vi "Temperatures.vi"(1 "Update Interval":i32=2 min=0 max=600, 2 "Control\nTemperature":sgl=-200.0 format="%.1f") -> (0 "DiodeTemp":dbl(slide) scale=-150.0..50.0)   [LabVIEW 2014]
uses:
  DetectorGlobals.vi
panel:
  in  "Tab Control":enum32{"CamTemp", "DewTemp", "Diode", "Temp4"}(tab)
  out "CamTemp Chart":dbl(graph)
  out "DewTemp Chart":dbl(graph)
  out "Diode Chart":dbl(graph)
  out "Temp4 Chart":dbl(graph)
  out "Utility Board\nInstalled":bool
  out "Temp 4":dbl(slide) scale=-150.0..50.0
  in  "Read Temps":bool
  out "Time1":dbl format="%.2f"
  out "refnum":refnum<file>
  in  "Log Data":bool
  in  "Read Heater":bool=TRUE caption="Read"
  out "Heater\nPower":dbl(knob) scale=0.0..3072.0
  out "DewTemp":dbl(slide) scale=-200.0..50.0
  out "CamTemp":dbl(slide) scale=-150.0..50.0
  in  "Set":bool
  # "C"
  # "sec"
  # "Degrees Celsius"
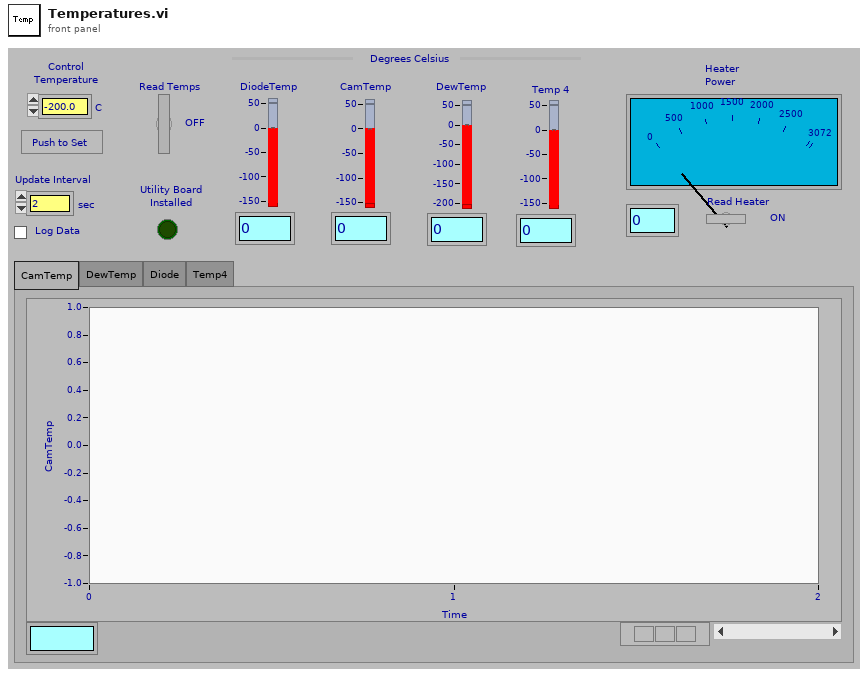
[diagram p1: front panel]
types:
  T1 = enum32{"not used", "PCI_BOARD", "TIMING_BOARD", "UTILITY_BOARD"}
  T2 = enum16{"open", "open or create", "create or replace", "create", "open (read only)"}
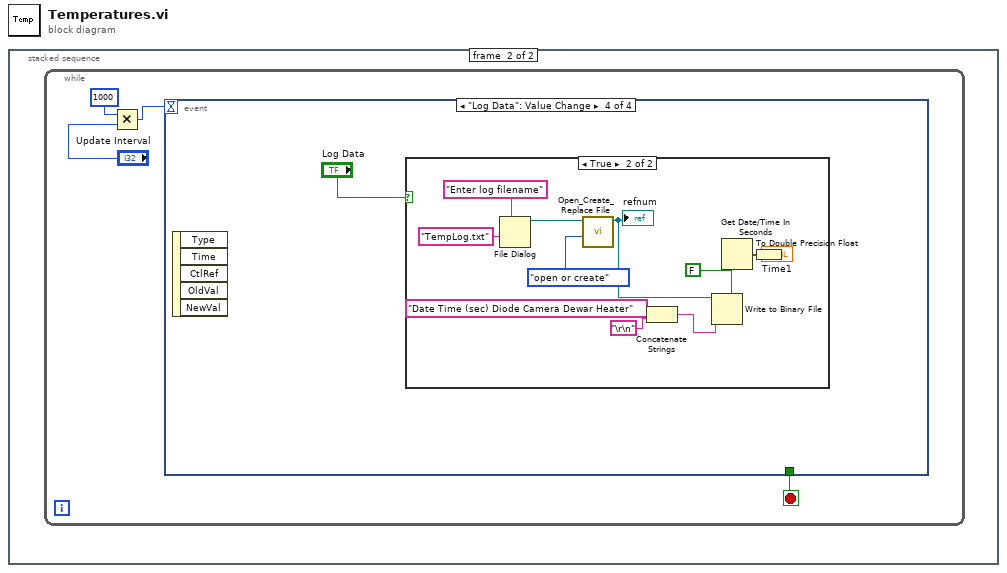
[diagram p0: block diagram]
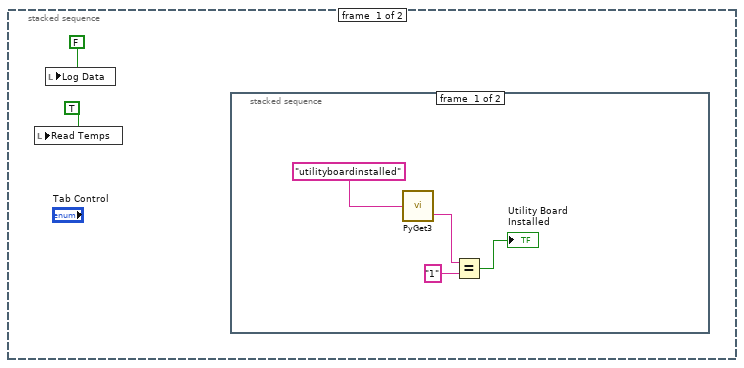
[diagram p2: hidden frame]
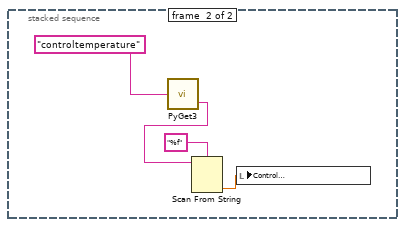
[diagram p3: hidden frame]
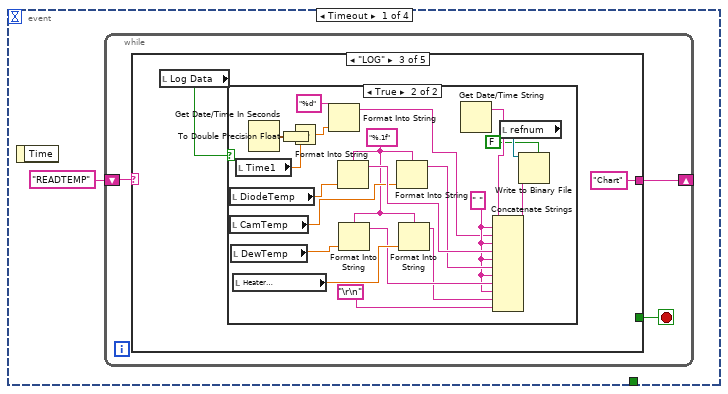
[diagram p4: hidden frame]
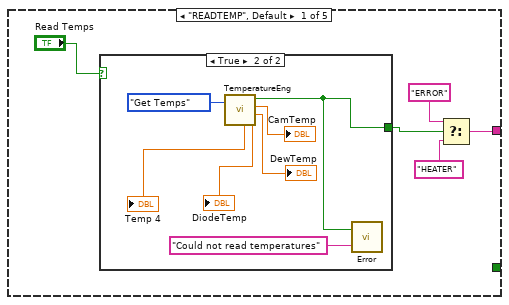
[diagram p5: hidden frame]
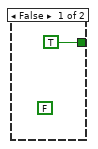
[diagram p6: hidden frame]
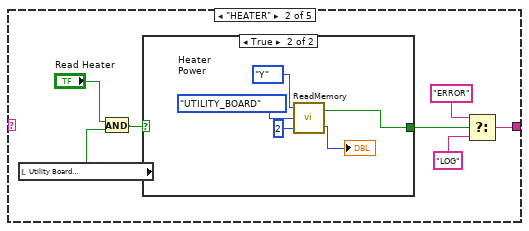
[diagram p7: hidden frame]
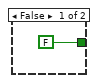
[diagram p8: hidden frame]
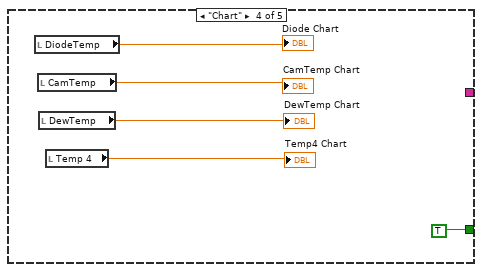
[diagram p10: hidden frame]
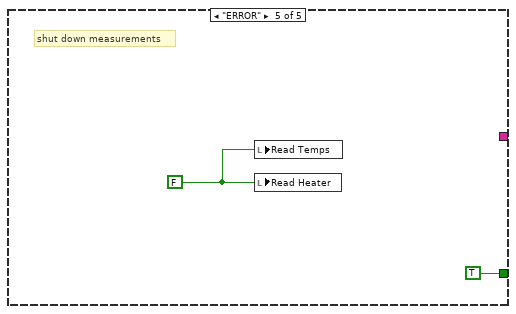
[diagram p11: hidden frame]
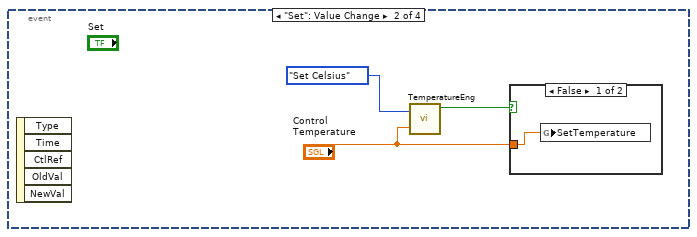
[diagram p12: hidden frame]
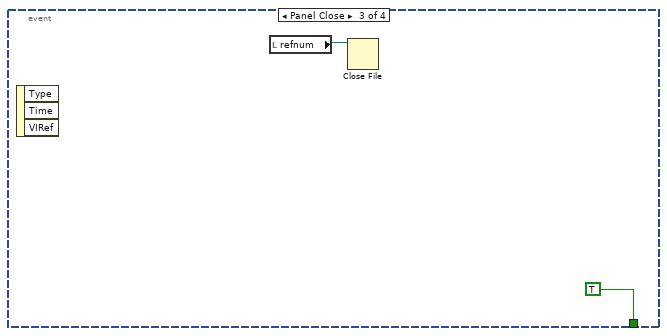
[diagram p14: hidden frame]
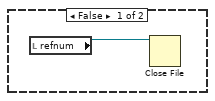
[diagram p15: hidden frame]
diagram:
  n1 = stacked-sequence {
    frame #0 {
      n2 = local write "Read Temps"(TRUE ("ReadTemps")) -> ()
      n3 = local write "Log Data"(FALSE ("Log Data")) -> ()
      n4 = stacked-sequence {
        frame #0 {
          n5 = call "PyGet3.vi"("Attribute"="utilityboardinstalled") -> ("Reply"=w5:string)  [unwired: 1 out]
          n6 = Equal?(x=w5, y="1") -> (x = y?=→"Utility Board\nInstalled":bool)
        }
        frame #1 {
          n7 = call "PyGet3.vi"("Attribute"="controltemperature") -> ("Reply"=w9:string)  [unwired: 1 out]
          n8 = Scan From String(format string="%f", input string=w9) -> (output 1=w7:dbl)  [unwired: 3 in, 3 out]
          n9 = local write "Control\nTemperature"(w7) -> ()
        }
      }
    }
    frame #1 {
      n10 = while {
        stop <- w11 stop-if-true
        n11 = Multiply(x=1000, y="Update Interval") -> (x*y=w13:i32)
        n12 = event shown="[3] \"Log Data\": Value Change" {
          selector: _ -> [_ _ _ _]
          dyn-events: _ -> [_ _ _ _]
          timeout: w13 -> [_ _ _ _]
          tunnel: [_ _ TRUE _] -> w11
          event Timeout {
            n13 = event-data() -> ()  [unwired: 1 in, 1 out]
            n14 = while {
              shift-right: [w18] -> _
              shift-left: "READTEMP" ("Error String") -> [w17]
              stop <- w16 stop-if-true
              n15 = case shown="\"LOG\"" w17 {
                tunnel: [w23 w38 "Chart" ("Error String") _ _] -> w18
                tunnel: [_ _ _ TRUE TRUE] -> w16
                frame "READTEMP", Default {
                  n16 = case shown="True" "Read Temps" {
                    tunnel: [TRUE w30] -> w22
                    frame False {
                      (unwired) FALSE ("Error")
                    }
                    frame True {
                      n17 = call "TemperatureEng.vi"("Action"=enum16{"Set Celsius", "Get Temps"}."Get Temps") -> ("Output3"=→"DiodeTemp":sgl, "Output2"=→"DewTemp":sgl, "Output1"=→"CamTemp":sgl, "Error"=w30:bool, "Output4"=→"Temp 4":sgl)  [unwired: 1 in]
                      n18 = call "Error.vi"("Error String"="Could not read temperatures", "Error In"=w30) -> ()  [unwired: 1 in, 1 out]
                    }
                  }
                  n19 = Select(t="ERROR" ("Error String"), s=w22, f="HEATER" ("Error String")) -> (s? t:f=w23:string)
                }
                frame "HEATER" {
                  n20 = local read "Utility Board\nInstalled"() -> (w32:bool)
                  n21 = And(x="Read Heater", y=w32) -> (x .and. y?=w34:bool)
                  n22 = case shown="True" w34 {
                    tunnel: [FALSE w40] -> w37
                    frame False {
                    }
                    frame True {
                      n23 = call "ReadMemory.vi"("Address"=2, "Board"=T1."UTILITY_BOARD", "Type"=enum16{"X", "Y", "P", "R", "D"}."Y") -> ("Value"=→"Heater\nPower":i32, "Error"=w40:bool)
                    }
                  }
                  n24 = Select(t="ERROR" ("Error String"), s=w37, f="LOG" ("Error String")) -> (s? t:f=w38:string)
                }
                frame "LOG" {
                  n25 = local read "Log Data"() -> (w46:bool)
                  n26 = case shown="True" w46 {
                    frame False {
                    }
                    frame True {
                      w52 = "%.1f" ("format string")
                      w59 = " " ("string")
                      n27 = local read "DiodeTemp"() -> (w65:dbl)
                      n28 = local read "CamTemp"() -> (w56:dbl)
                      n29 = local read "DewTemp"() -> (w64:dbl)
                      n30 = local read "Heater\nPower"() -> (w63:dbl)
                      n31 = local read "Time1"() -> (w54:dbl)
                      n32 = Get Date/Time In Seconds() -> (seconds since 1Jan1904=w48:timestamp)
                      n33 = To Double Precision Float(number=w48) -> (double precision float=w53:dbl)
                      n34 = Subtract(x=w53, y=w54) -> (x-y=w51:dbl)
                      n35 = Format Into String(format string="%d", w51) -> (resulting string=w50:string)  [unwired: 2 in, 1 out]
                      n36 = Format Into String(format string=w52, w65) -> (resulting string=w62:string)  [unwired: 2 in, 1 out]
                      n37 = Format Into String(format string=w52, w64) -> (resulting string=w60:string)  [unwired: 2 in, 1 out]
                      n38 = Format Into String(format string=w52, w56) -> (resulting string=w61:string)  [unwired: 2 in, 1 out]
                      n39 = Format Into String(format string=w52, w63) -> (resulting string=w58:string)  [unwired: 2 in, 1 out]
                      n40 = Get Date/Time String() -> (date string=w55:string)  [unwired: 3 in, 1 out]
                      n41 = Concatenate Strings(w55, w59, w50, w59, w62, w59, w61, w59, w60, w59, w58, "\r\n") -> (w66:string)
                      n42 = local read "refnum"() -> (w67:refnum<file>)
                      n43 = Write to Binary File(file (use dialog)=w67, data=w66, 5:FALSE ("prepend array or string size? (T)")) -> ()  [unwired: 3 in, 3 out]
                    }
                  }
                }
                frame "Chart" {
                  n44 = local read "DiodeTemp"() -> (→"Diode Chart":dbl)
                  n45 = local read "CamTemp"() -> (→"CamTemp Chart":dbl)
                  n46 = local read "DewTemp"() -> (→"DewTemp Chart":dbl)
                  n47 = local read "Temp 4"() -> (→"Temp4 Chart":dbl)
                }
                frame "ERROR" {
                  w73 = FALSE
                  # "shut down measurements"
                  n48 = local write "Read Temps"(w73) -> ()
                  n49 = local write "Read Heater"(w73) -> ()
                }
              }
            }
          }
          event "Set": Value Change {
            n50 = event-data() -> ()  [unwired: 1 in, 5 out]
            n51 = call "TemperatureEng.vi"("Set Temperature"="Control\nTemperature", "Action"=enum16{"Set Celsius", "Get Temps"}."Set Celsius") -> ("Error"=w75:bool)  [unwired: 4 out]
            n52 = case shown="False" w75 {
              tunnel: "Control\nTemperature" -> [w78 _]
              frame False {
                n53 = global write "DetectorGlobals.vi" "SetTemperature"(w78) -> ()
              }
              frame True {
              }
            }
          }
          event Panel Close {
            n54 = event-data() -> ()  [unwired: 1 in, 3 out]
            n55 = local read "refnum"() -> (w79:refnum<file>)
            n56 = Close File(refnum=w79) -> ()  [unwired: 1 in, 2 out]
          }
          event "Log Data": Value Change {
            n57 = event-data() -> ()  [unwired: 1 in, 5 out]
            n58 = case shown="True" "Log Data" {
              frame False {
                n59 = local read "refnum"() -> (w82:refnum<file>)
                n60 = Close File(refnum=w82) -> ()  [unwired: 1 in, 2 out]
              }
              frame True {
                n61 = File Dialog(7:"Enter log filename" ("prompt"), 9:"TempLog.txt" ("default name")) -> (3:w92:path)  [unwired: 5 in, 3 out]
                n62 = call <vilib>:"Open_Create_Replace File.vi"("function (open:0)"=T2."open or create", "file path"=w92) -> ("refnum"=w89:refnum<file>)  [unwired: 6 in, 3 out]
                "refnum" <- w89
                n63 = Concatenate Strings("Date Time (sec) Diode Camera Dewar Heater" ("default name"), "\r\n") -> (w86:string)
                n64 = Write to Binary File(file (use dialog)=w89, data=w86, 5:FALSE ("prepend array or string size? (T)")) -> ()  [unwired: 3 in, 3 out]
                n65 = Get Date/Time In Seconds() -> (seconds since 1Jan1904=w84:timestamp)
                n66 = To Double Precision Float(number=w84) -> (double precision float=→"Time1":dbl)
              }
            }
          }
        }
      }
    }
  }
